vi "sortMFCs.vi"(11 "MFCs":T1[](array[typedef])) -> (0 "InUseMFCsdescending":T1[](array[typedef]), 1 "InUseMFCsascending":T1[](array[typedef]), 2 "notInUseMFCsdescending":T1[](array[typedef]), 3 "notInUseMFCsascending":T1[](array[typedef]))   [LabVIEW 2016]
uses:
  MFCdescription.ctl
  MFCcapability.ctl
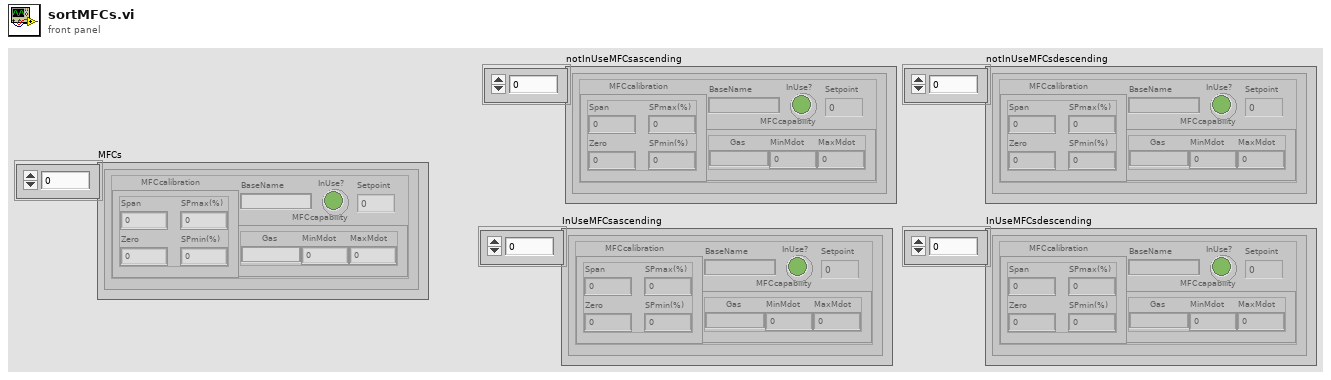
[diagram p1: front panel]
types:
  T1 = typedef "MFCdescription.ctl" = cluster{"BaseName":string, "MFCcalibration":cluster{"Span":dbl, "Zero":dbl, "SPmin(%)":dbl, "SPmax(%)":dbl}, "MFCcapability":T2, "InUse?":bool, "Setpoint":dbl}
  T2 = typedef "MFCcapability.ctl" = cluster{"Gas":string, "MinMdot":dbl, "MaxMdot":dbl}
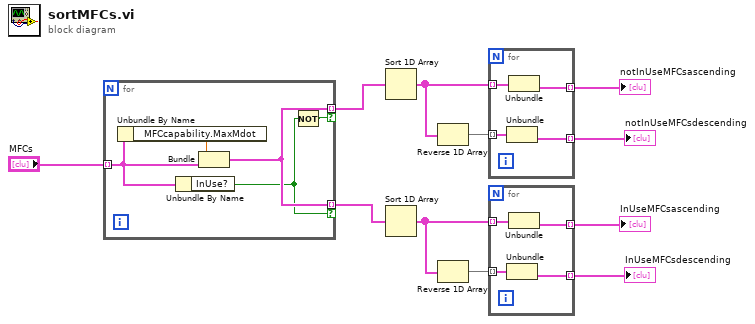
[diagram p0: block diagram]
diagram:
  n1 = for {
    tunnel: "MFCs" -> [w15] mode=indexing
    tunnel: [w14] -> w6 mode=indexing if=w13
    tunnel: [w14] -> w1 mode=indexing if=w12
    n2 = Unbundle By Name(w15) -> ("MFCcapability.MaxMdot"=w16:dbl)
    n3 = Unbundle By Name(w15) -> ("InUse?"=w13:bool)
    n4 = Bundle("MaxMdot"=w16, "Cluster"=w15) -> (w14:cluster{"MaxMdot":dbl, "Cluster":T1})  [unwired: 1 in]
    n5 = Not(x=w13) -> (.not. x?=w12:bool)
  }
  n6 = Sort 1D Array(array=w1) -> (sorted array=w4:cluster{"MaxMdot":dbl, "Cluster":T1}[])
  n7 = Sort 1D Array(array=w6) -> (sorted array=w9:cluster{"MaxMdot":dbl, "Cluster":T1}[])
  n8 = Reverse 1D Array(array=w4) -> (reversed array=w3:cluster{"MaxMdot":dbl, "Cluster":T1}[])
  n9 = Reverse 1D Array(array=w9) -> (reversed array=w10:cluster{"MaxMdot":dbl, "Cluster":T1}[])
  n10 = for {
    tunnel: w4 -> [w20] mode=indexing
    tunnel: [w19] -> w5 mode=indexing
    tunnel: w3 -> [w18] mode=indexing
    tunnel: [w17] -> w2 mode=indexing
    n11 = Unbundle(w18) -> ("Cluster"=w17:T1)  [unwired: 1 out]
    n12 = Unbundle(w20) -> ("Cluster"=w19:T1)  [unwired: 1 out]
  }
  "notInUseMFCsdescending" <- w2
  "notInUseMFCsascending" <- w5
  n13 = for {
    tunnel: w9 -> [w24] mode=indexing
    tunnel: [w23] -> w8 mode=indexing
    tunnel: w10 -> [w22] mode=indexing
    tunnel: [w21] -> w11 mode=indexing
    n14 = Unbundle(w22) -> ("Cluster"=w21:T1)  [unwired: 1 out]
    n15 = Unbundle(w24) -> ("Cluster"=w23:T1)  [unwired: 1 out]
  }
  "InUseMFCsdescending" <- w11
  "InUseMFCsascending" <- w8
